vi "MotorAlltoZero.vi"(11 "状态输入":refnum<vi>) -> ()   [LabVIEW 2018]
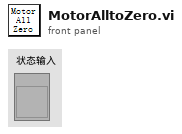
[diagram p1: front panel]
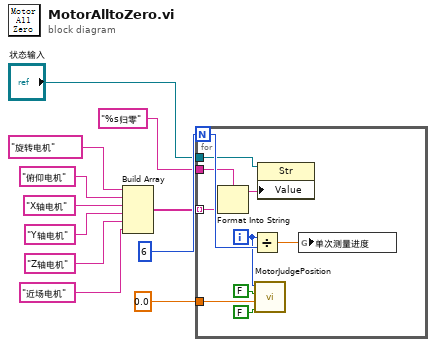
[diagram p0: block diagram]
diagram:
  n1 = Build Array("旋转电机", "俯仰电机", "X轴电机", "Y轴电机", "Z轴电机", "近场电机") -> (w3:string[])
  n2 = for {
    N: 6 -> [w21]
    tunnel: 0.0 ("位置") -> [w17]
    tunnel: w3 -> [w14] mode=indexing
    tunnel: "%s归零" ("格式字符串") -> [w15]
    tunnel: "状态输入" -> [w13]
    i -> [w19]
    n3 = Format Into String(format string=w15, w14) -> (resulting string=w12:string)  [unwired: 2 in, 1 out]
    n4 = Divide(x=w19, y=w21) -> (x/y=w20:dbl)
    n5 = call "MotorJudgePosition.vi"("是否需要测量进度"=FALSE, "位置"=w17, "直线电机？"=FALSE, "axis"=w19) -> ()  [unwired: 2 in, 1 out]
    n6 = property class="Str"(reference=w13, "Value"=w12) -> ()  [unwired: 1 in, 2 out]
    n7 = global write "globalMessage.vi" "单次测量进度"(w20) -> ()
  }
